vi "Exercise 10.3.vi"() -> ()   [LabVIEW 2010]
panel:
  in  "Walk Request":bool
  out "Walk Sign":bool
  out "Green":bool
  out "Yellow":bool
  out "Red":bool
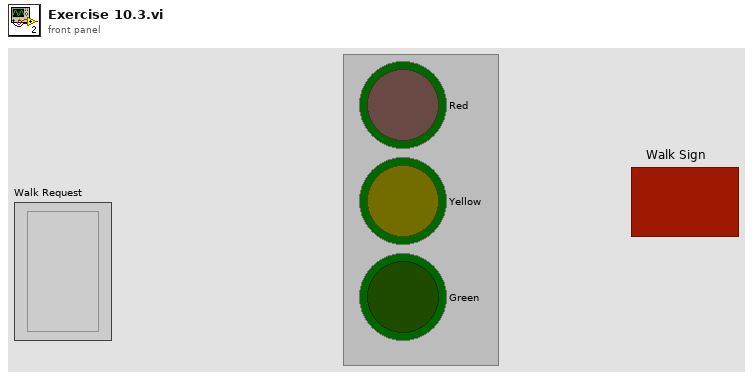
[diagram p1: front panel]
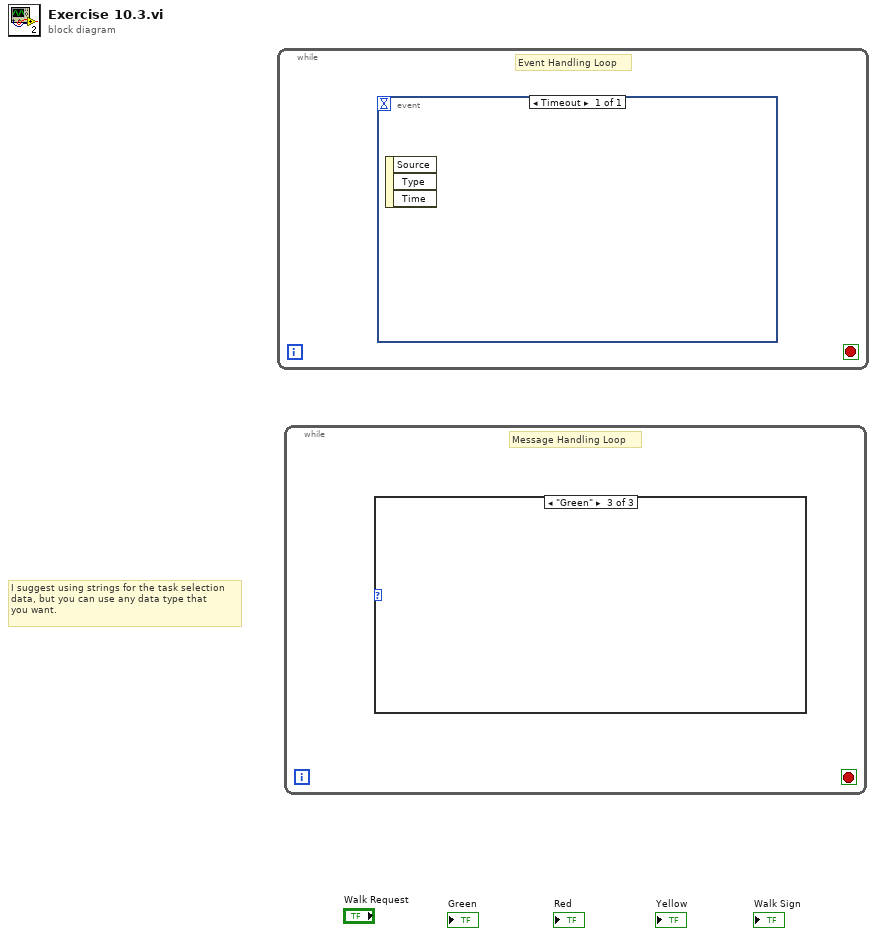
[diagram p0: block diagram]
diagram:
  # "I suggest using strings for the task selection\ndata, but you can use any data type that\nyou want."
  n1 = while {
    stop <- _ stop-if-true
    # "Event Handling Loop"
    n2 = event shown="[0] Timeout" {
      selector: _ -> [_]
      dyn-events: _ -> [_]
      timeout: _ -> [_]
      event Timeout {
        n3 = event-data() -> ()  [unwired: 1 in, 3 out]
      }
    }
  }
  n4 = while {
    stop <- _ stop-if-true
    # "Message Handling Loop"
    n5 = case shown="\"Green\"" {
      selector: _ -> [_ _ _]
      frame "Red", Default {
      }
      frame "Yellow" {
      }
      frame "Green" {
      }
    }
  }
